vi "RC_test_reader.vi"(8 "error in (no error)":errorcluster, 9 "Motors IDs Found":u8[](array[numeric]), 10 "Read positions (dyn)":dbl[](array[numeric]), 11 "VISA Refnum in":refnum<visa-resource-name>) -> (0 "error out":errorcluster[](array[cluster]), 2 "Dynamixel Positions (deg)":dbl[](array[numeric]), 3 "Read positions latest (dyn)":dbl[](array[numeric]))   [LabVIEW 2013]
doc: "This VI takes an array of motor IDs and reads the position of each one. It outputs as both raw values and as degrees.\n\nIt's set up for the SAIL Dynamixels, because it scales by 360/1200. We're still investigating whether the rudder has different units."
uses:
  <instrlib>/Dynamixel Motor/Dynamixel Motor.lvlib
panel:
  in  "Rudder ID":i8=127
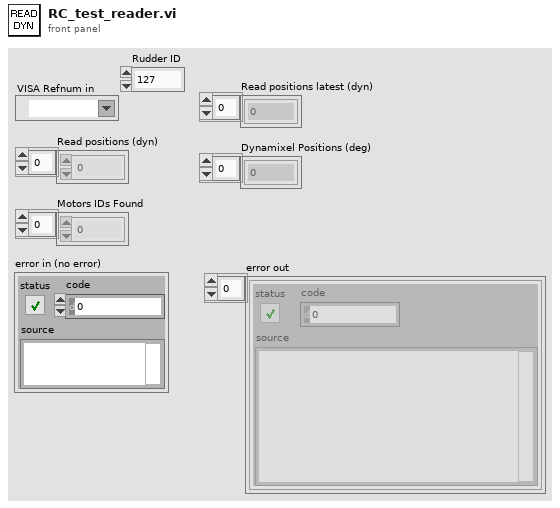
[diagram p1: front panel]
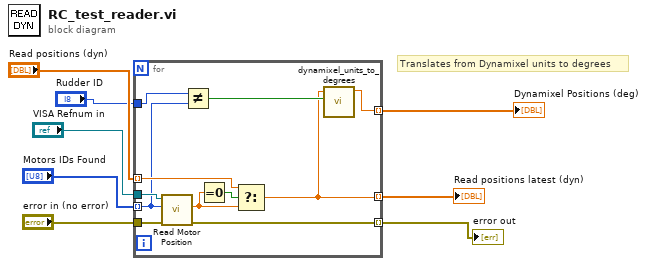
[diagram p0: block diagram]
diagram:
  # "Translates from Dynamixel units to degrees"
  n1 = for {
    tunnel: "VISA Refnum in" -> [w19]
    tunnel: "Motors IDs Found" -> [w13] mode=indexing
    tunnel: "error in (no error)" -> [w18]
    tunnel: [w17] -> w7 mode=indexing
    tunnel: "Read positions (dyn)" -> [w14] mode=indexing
    tunnel: "Rudder ID" -> [w12]
    tunnel: [w10] -> w2 mode=indexing
    tunnel: [w9] -> w1 mode=indexing
    n2 = call <instrlib>:"Read Motor Position.vi"("error in (no error)"=w18, "Motor ID (0)"=w13, "VISA resource name"=w19) -> ("error out"=w17:errorcluster, "Position (deg)"=w15:dbl)  [unwired: 6 in, 1 out]
    n3 = Not Equal?(x=w12, y=w13) -> (x != y?=w11:bool)
    n4 = Equal To 0?(x=w15) -> (x = 0?=w16:bool)
    n5 = Select(t=w14, s=w16, f=w15) -> (s? t:f=w10:dbl)
    n6 = call "dynamixel_units_to_degrees.vi"("MX Motor? (T)"=w11, "Dynamixel Input"=w10) -> ("Degrees"=w9:dbl)  [unwired: 8 in, 1 out]
  }
  "Read positions latest (dyn)" <- w2
  "Dynamixel Positions (deg)" <- w1
  "error out" <- w7
